vi "config_ini.vi"(11 "Path":path) -> ()   [LabVIEW 2013]
uses:
  <vilib>/Utility/config.llb/Read Key (Boolean).vi
  <vilib>/Utility/config.llb/Read Key (Double).vi
  FT_HMI.llb/GLOBAL_PUMPS_PARAMS.vi
  <vilib>/Utility/config.llb/NI_LVConfig.lvlib
panel:
  out "PUMPS_PARAMS":T1
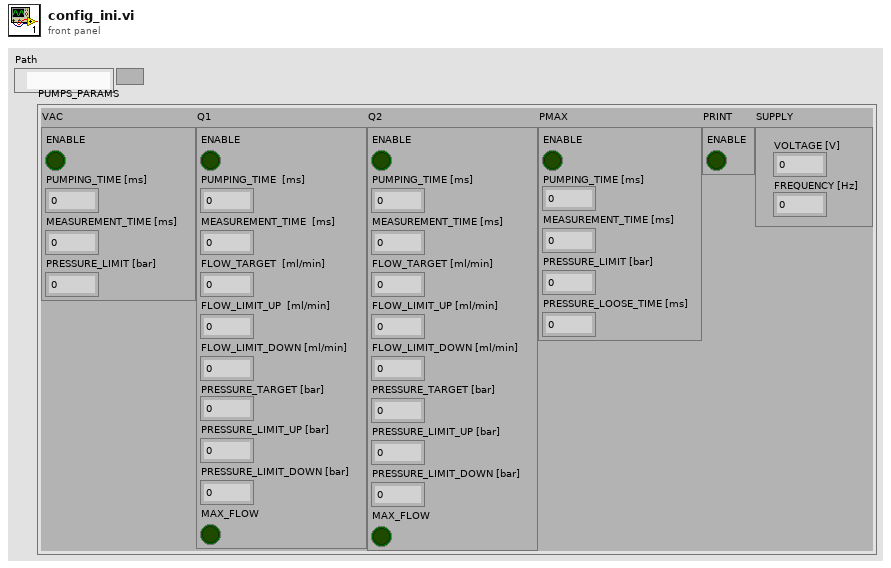
[diagram p1: front panel]
types:
  T1 = cluster{"VAC":cluster{"ENABLE":bool, "PUMPING_TIME [ms]":dbl, "MEASUREMENT_TIME [ms]":dbl, "PRESSURE_LIMIT [bar]":sgl}, "Q1":cluster{"ENABLE":bool, "PUMPING_TIME  [ms]":dbl, "MEASUREMENT_TIME  [ms]":sgl, "FLOW_TARGET  [ml/min]":sgl, "FLOW_LIMIT_UP  [ml/min]":sgl, "FLOW_LIMIT_DOWN [ml/min]":sgl, "PRESSURE_TARGET [bar]":sgl, "PRESSURE_LIMIT_UP [bar]":sgl, "PRESSURE_LIMIT_DOWN [bar]":sgl, "MAX_FLOW":bool}, "Q2":cluster{"ENABLE":bool, "PUMPING_TIME [ms]":dbl, "MEASUREMENT_TIME [ms]":dbl, "FLOW_TARGET [ml/min]":sgl, "FLOW_LIMIT_UP [ml/min]":sgl, "FLOW_LIMIT_DOWN [ml/min]":sgl, "PRESSURE_TARGET [bar]":sgl, "PRESSURE_LIMIT_UP [bar]":sgl, "PRESSURE_LIMIT_DOWN [bar]":sgl, "MAX_FLOW":bool}, "PMAX":cluster{"ENABLE":bool, "PUMPING_TIME [ms]":dbl, "MEASUREMENT_TIME [ms]":dbl, "PRESSURE_LIMIT [bar]":sgl, "PRESSURE_LOOSE_TIME [ms]":sgl}, "PRINT":cluster{"ENABLE":bool}, "SUPPLY":cluster{"VOLTAGE [V]":dbl, "FREQUENCY [Hz]":dbl}}
  T2 = typedef "NI_LVConfig.lvlib/Config Data RefNum.ctl" = refnum<k1>
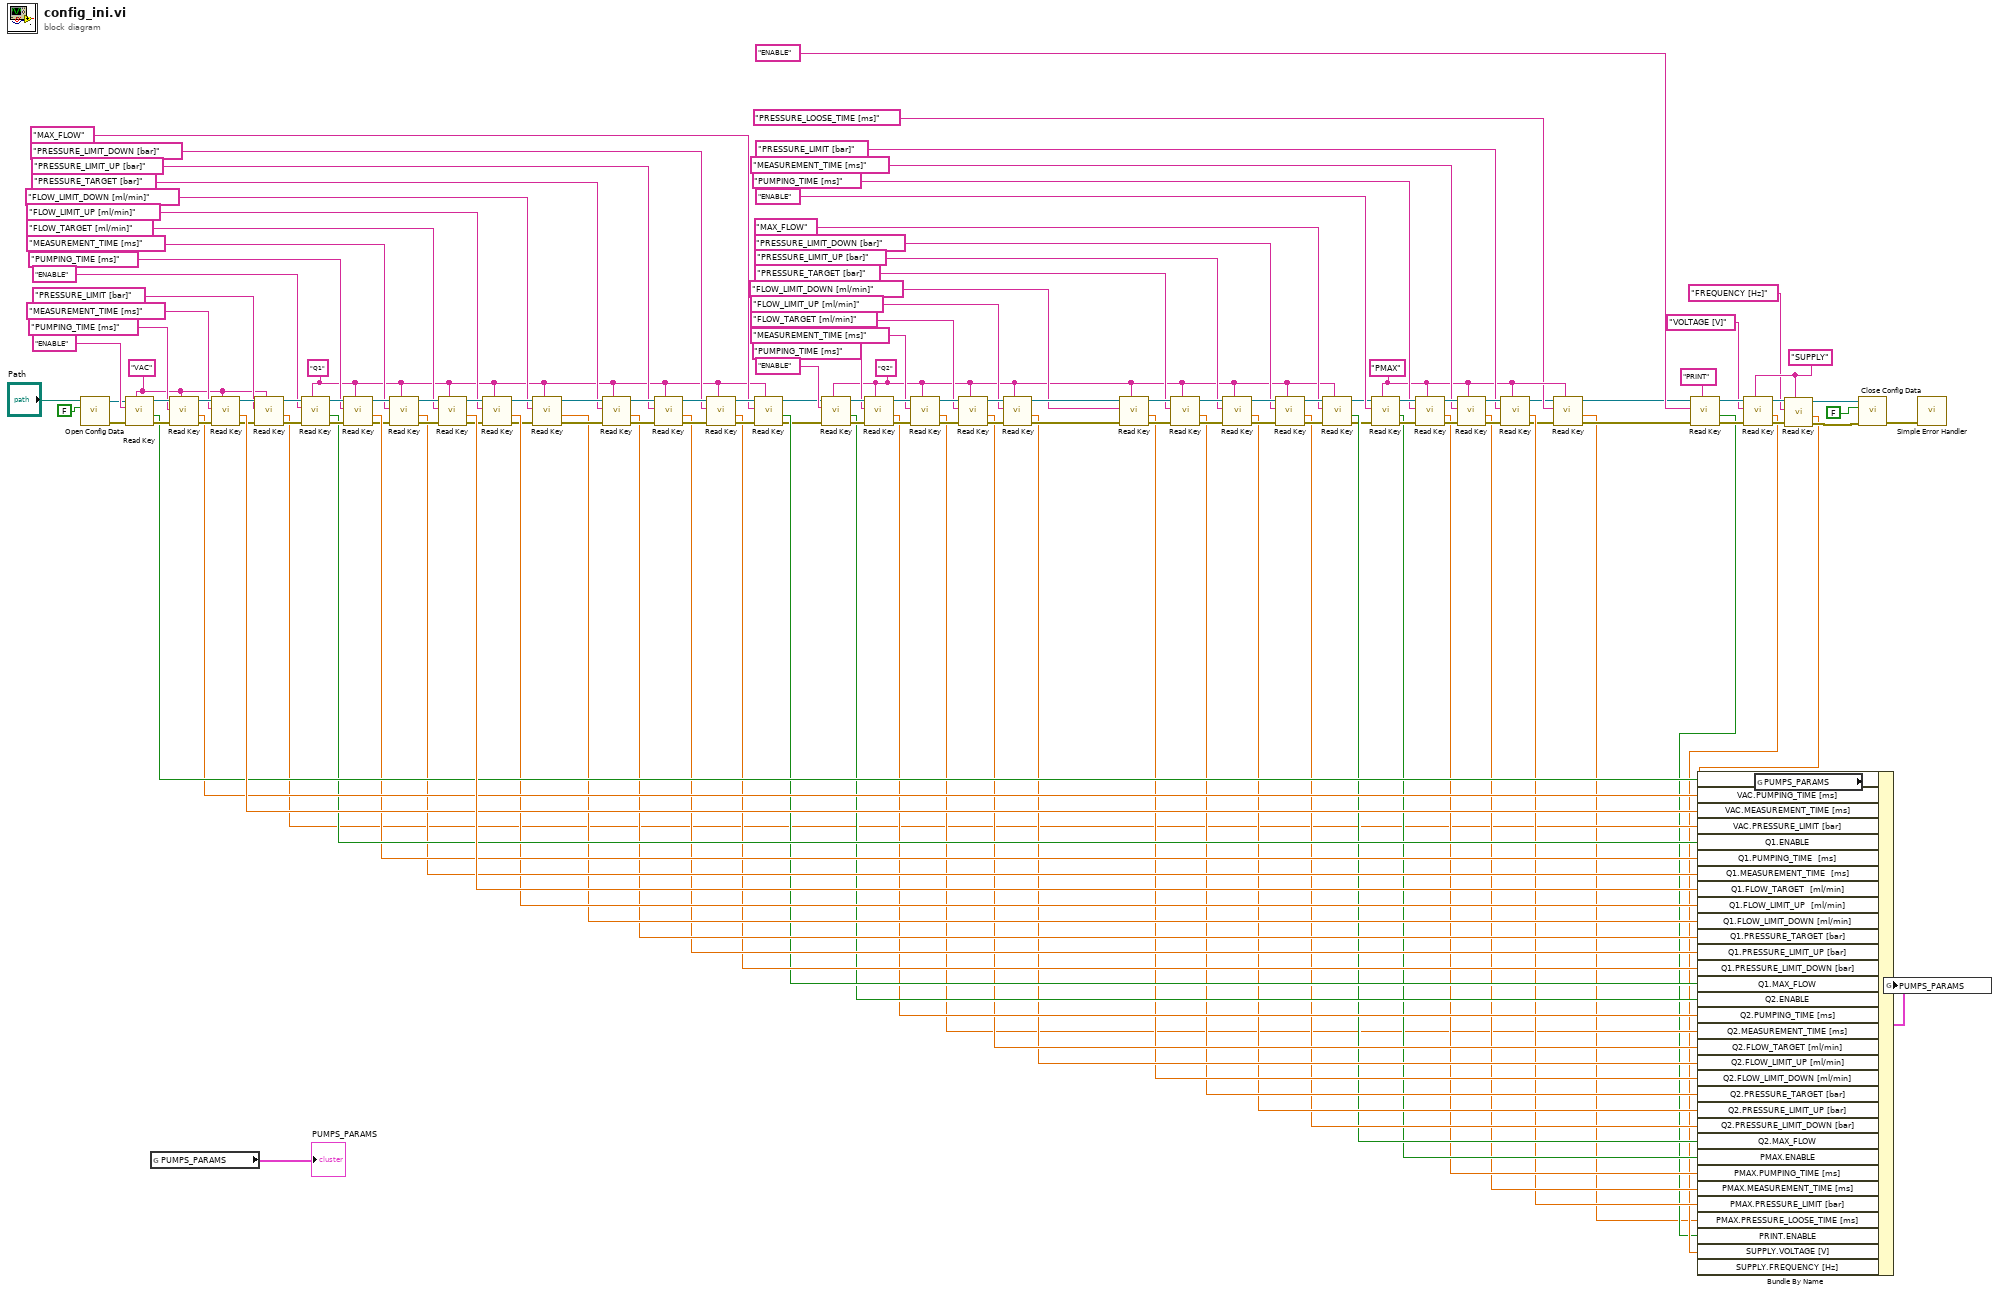
[diagram p0: block diagram]
diagram:
  w15 = "SUPPLY" ("section")
  w5 = "PMAX" ("section")
  w52 = "Q2" ("section")
  w81 = "Q1" ("section")
  w122 = "VAC" ("section")
  n1 = call <vilib>:"Open Config Data.vi"("create file if necessary (T)"=FALSE ("create file if necessary? (T)"), "configuration file path"="Path") -> ("error out"=w126:errorcluster, "refnum"=w125:T2)  [unwired: 7 in, 1 out]
  n2 = call-poly <vilib>:"Read Key.vi"("section"=w122, "error in (no error)"=w126, "key"="ENABLE" ("Key 1"), "refnum"=w125) -> ("error out"=w140:errorcluster, "value"=w116:bool, "refnum out"=w138:T2)  [unwired: 1 in, 4 out]
  n3 = global read "GLOBAL_PUMPS_PARAMS.vi" "PUMPS_PARAMS"() -> (→"PUMPS_PARAMS":T1)
  n4 = call-poly <vilib>:"Read Key.vi"("section"=w122, "error in (no error)"=w140, "key"="PUMPING_TIME [ms]" ("Key 2"), "refnum"=w138) -> ("error out"=w135:errorcluster, "value"=w115:dbl, "refnum out"=w136:T2)  [unwired: 1 in, 4 out]
  n5 = call-poly <vilib>:"Read Key.vi"("section"=w122, "error in (no error)"=w135, "key"="MEASUREMENT_TIME [ms]" ("Key 3"), "refnum"=w136) -> ("error out"=w139:errorcluster, "value"=w142:dbl, "refnum out"=w137:T2)  [unwired: 4 in, 1 out]
  n6 = call-poly <vilib>:"Read Key.vi"("section"=w122, "error in (no error)"=w139, "key"="PRESSURE_LIMIT [bar]" ("Key 4"), "refnum"=w137) -> ("error out"=w134:errorcluster, "value"=w11:dbl, "refnum out"=w133:T2)  [unwired: 2 in, 3 out]
  n7 = call-poly <vilib>:"Read Key.vi"("section"=w81, "error in (no error)"=w134, "key"="ENABLE" ("Key 5"), "refnum"=w133) -> ("error out"=w120:errorcluster, "value"=w114:bool, "refnum out"=w121:T2)  [unwired: 2 in, 3 out]
  n8 = call-poly <vilib>:"Read Key.vi"("section"=w81, "error in (no error)"=w120, "key"="PUMPING_TIME [ms]" ("Key 2"), "refnum"=w121) -> ("error out"=w107:errorcluster, "value"=w113:dbl, "refnum out"=w112:T2)  [unwired: 2 in, 3 out]
  n9 = call-poly <vilib>:"Read Key.vi"("section"=w81, "error in (no error)"=w107, "key"="MEASUREMENT_TIME [ms]" ("Key 3"), "refnum"=w112) -> ("error out"=w108:errorcluster, "value"=w103:dbl, "refnum out"=w111:T2)  [unwired: 2 in, 3 out]
  n10 = call-poly <vilib>:"Read Key.vi"("section"=w81, "error in (no error)"=w108, "key"="FLOW_TARGET [ml/min]" ("Key 3"), "refnum"=w111) -> ("error out"=w109:errorcluster, "value"=w143:dbl, "refnum out"=w110:T2)  [unwired: 2 in, 3 out]
  n11 = call-poly <vilib>:"Read Key.vi"("section"=w81, "error in (no error)"=w109, "key"="FLOW_LIMIT_UP [ml/min]" ("Key 3"), "refnum"=w110) -> ("error out"=w101:errorcluster, "value"=w102:dbl, "refnum out"=w96:T2)  [unwired: 2 in, 3 out]
  n12 = call-poly <vilib>:"Read Key.vi"("section"=w81, "error in (no error)"=w101, "key"="FLOW_LIMIT_DOWN [ml/min]" ("Key 3"), "refnum"=w96) -> ("error out"=w100:errorcluster, "value"=w86:dbl, "refnum out"=w95:T2)  [unwired: 2 in, 3 out]
  n13 = call-poly <vilib>:"Read Key.vi"("section"=w81, "error in (no error)"=w100, "key"="PRESSURE_TARGET [bar]" ("Key 3"), "refnum"=w95) -> ("error out"=w99:errorcluster, "value"=w85:dbl, "refnum out"=w94:T2)  [unwired: 2 in, 3 out]
  n14 = call-poly <vilib>:"Read Key.vi"("section"=w81, "error in (no error)"=w99, "key"="PRESSURE_LIMIT_UP [bar]" ("Key 3"), "refnum"=w94) -> ("error out"=w98:errorcluster, "value"=w84:dbl, "refnum out"=w93:T2)  [unwired: 2 in, 3 out]
  n15 = call-poly <vilib>:"Read Key.vi"("section"=w81, "error in (no error)"=w98, "key"="PRESSURE_LIMIT_DOWN [bar]" ("Key 3"), "refnum"=w93) -> ("error out"=w97:errorcluster, "value"=w83:dbl, "refnum out"=w92:T2)  [unwired: 2 in, 3 out]
  n16 = call-poly <vilib>:"Read Key.vi"("section"=w81, "error in (no error)"=w97, "key"="MAX_FLOW" ("Key 5"), "refnum"=w92) -> ("error out"=w51:errorcluster, "value"=w82:bool, "refnum out"=w50:T2)  [unwired: 2 in, 3 out]
  n17 = call-poly <vilib>:"Read Key.vi"("section"=w52, "error in (no error)"=w51, "key"="ENABLE" ("Key 5"), "refnum"=w50) -> ("error out"=w78:errorcluster, "value"=w49:bool, "refnum out"=w79:T2)  [unwired: 2 in, 3 out]
  n18 = call-poly <vilib>:"Read Key.vi"("section"=w52, "error in (no error)"=w78, "key"="PUMPING_TIME [ms]" ("Key 2"), "refnum"=w79) -> ("error out"=w71:errorcluster, "value"=w48:dbl, "refnum out"=w76:T2)  [unwired: 2 in, 3 out]
  n19 = call-poly <vilib>:"Read Key.vi"("section"=w52, "error in (no error)"=w71, "key"="MEASUREMENT_TIME [ms]" ("Key 3"), "refnum"=w76) -> ("error out"=w72:errorcluster, "value"=w13:dbl, "refnum out"=w75:T2)  [unwired: 2 in, 3 out]
  n20 = call-poly <vilib>:"Read Key.vi"("section"=w52, "error in (no error)"=w72, "key"="FLOW_TARGET [ml/min]" ("Key 3"), "refnum"=w75) -> ("error out"=w73:errorcluster, "value"=w47:dbl, "refnum out"=w74:T2)  [unwired: 2 in, 3 out]
  n21 = call-poly <vilib>:"Read Key.vi"("section"=w52, "error in (no error)"=w73, "key"="FLOW_LIMIT_UP [ml/min]" ("Key 3"), "refnum"=w74) -> ("error out"=w67:errorcluster, "value"=w46:dbl, "refnum out"=w62:T2)  [unwired: 2 in, 3 out]
  n22 = call-poly <vilib>:"Read Key.vi"("section"=w52, "error in (no error)"=w67, "key"="FLOW_LIMIT_DOWN [ml/min]" ("Key 3"), "refnum"=w62) -> ("error out"=w66:errorcluster, "value"=w45:dbl, "refnum out"=w61:T2)  [unwired: 2 in, 3 out]
  n23 = call-poly <vilib>:"Read Key.vi"("section"=w52, "error in (no error)"=w66, "key"="PRESSURE_TARGET [bar]" ("Key 3"), "refnum"=w61) -> ("error out"=w65:errorcluster, "value"=w44:dbl, "refnum out"=w60:T2)  [unwired: 2 in, 3 out]
  n24 = call-poly <vilib>:"Read Key.vi"("section"=w52, "error in (no error)"=w65, "key"="PRESSURE_LIMIT_UP [bar]" ("Key 3"), "refnum"=w60) -> ("error out"=w64:errorcluster, "value"=w43:dbl, "refnum out"=w59:T2)  [unwired: 2 in, 3 out]
  n25 = call-poly <vilib>:"Read Key.vi"("section"=w52, "error in (no error)"=w64, "key"="PRESSURE_LIMIT_DOWN [bar]" ("Key 3"), "refnum"=w59) -> ("error out"=w63:errorcluster, "value"=w42:dbl, "refnum out"=w58:T2)  [unwired: 2 in, 3 out]
  n26 = call-poly <vilib>:"Read Key.vi"("section"=w52, "error in (no error)"=w63, "key"="MAX_FLOW" ("Key 5"), "refnum"=w58) -> ("error out"=w24:errorcluster, "value"=w41:bool, "refnum out"=w23:T2)  [unwired: 2 in, 3 out]
  n27 = call-poly <vilib>:"Read Key.vi"("section"=w5, "error in (no error)"=w24, "key"="ENABLE" ("Key 1"), "refnum"=w23) -> ("error out"=w40:errorcluster, "value"=w30:bool, "refnum out"=w38:T2)  [unwired: 1 in, 4 out]
  n28 = call-poly <vilib>:"Read Key.vi"("section"=w5, "error in (no error)"=w40, "key"="PUMPING_TIME [ms]" ("Key 2"), "refnum"=w38) -> ("error out"=w35:errorcluster, "value"=w29:dbl, "refnum out"=w36:T2)  [unwired: 1 in, 4 out]
  n29 = call-poly <vilib>:"Read Key.vi"("section"=w5, "error in (no error)"=w35, "key"="MEASUREMENT_TIME [ms]" ("Key 3"), "refnum"=w36) -> ("error out"=w39:errorcluster, "value"=w28:dbl, "refnum out"=w37:T2)  [unwired: 4 in, 1 out]
  n30 = call-poly <vilib>:"Read Key.vi"("section"=w5, "error in (no error)"=w39, "key"="PRESSURE_LIMIT [bar]" ("Key 4"), "refnum"=w37) -> ("error out"=w1:errorcluster, "value"=w27:dbl, "refnum out"=w2:T2)  [unwired: 2 in, 3 out]
  n31 = call-poly <vilib>:"Read Key.vi"("section"=w5, "error in (no error)"=w1, "key"="PRESSURE_LOOSE_TIME [ms]" ("Key 4"), "refnum"=w2) -> ("error out"=w7:errorcluster, "value"=w3:dbl, "refnum out"=w6:T2)  [unwired: 2 in, 3 out]
  n32 = call-poly <vilib>:"Read Key.vi"("section"="PRINT", "error in (no error)"=w7, "key"="ENABLE" ("Key 5"), "refnum"=w6) -> ("error out"=w22:errorcluster, "value"=w8:bool, "refnum out"=w21:T2)  [unwired: 1 in, 4 out]
  n33 = call-poly <vilib>:"Read Key.vi"("section"=w15, "error in (no error)"=w22, "key"="VOLTAGE [V]" ("Key 4"), "refnum"=w21) -> ("error out"=w19:errorcluster, "value"=w9:dbl, "refnum out"=w17:T2)  [unwired: 4 in, 1 out]
  n34 = global read "GLOBAL_PUMPS_PARAMS.vi" "PUMPS_PARAMS"() -> (w118:T1)
  n35 = call-poly <vilib>:"Read Key.vi"("section"=w15, "error in (no error)"=w19, "key"="FREQUENCY [Hz]" ("Key 3"), "refnum"=w17) -> ("error out"=w18:errorcluster, "value"=w10:dbl, "refnum out"=w16:T2)  [unwired: 4 in, 1 out]
  n36 = Bundle By Name(cluster=w118, "VAC.ENABLE"=w116, "VAC.PUMPING_TIME [ms]"=w115, "VAC.MEASUREMENT_TIME [ms]"=w142, "VAC.PRESSURE_LIMIT [bar]"=w11, "Q1.ENABLE"=w114, "Q1.PUMPING_TIME  [ms]"=w113, "Q1.MEASUREMENT_TIME  [ms]"=w103, "Q1.FLOW_TARGET  [ml/min]"=w143, "Q1.FLOW_LIMIT_UP  [ml/min]"=w102, "Q1.FLOW_LIMIT_DOWN [ml/min]"=w86, "Q1.PRESSURE_TARGET [bar]"=w85, "Q1.PRESSURE_LIMIT_UP [bar]"=w84, "Q1.PRESSURE_LIMIT_DOWN [bar]"=w83, "Q1.MAX_FLOW"=w82, "Q2.ENABLE"=w49, "Q2.PUMPING_TIME [ms]"=w48, "Q2.MEASUREMENT_TIME [ms]"=w13, "Q2.FLOW_TARGET [ml/min]"=w47, "Q2.FLOW_LIMIT_UP [ml/min]"=w46, "Q2.FLOW_LIMIT_DOWN [ml/min]"=w45, "Q2.PRESSURE_TARGET [bar]"=w44, "Q2.PRESSURE_LIMIT_UP [bar]"=w43, "Q2.PRESSURE_LIMIT_DOWN [bar]"=w42, "Q2.MAX_FLOW"=w41, "PMAX.ENABLE"=w30, "PMAX.PUMPING_TIME [ms]"=w29, "PMAX.MEASUREMENT_TIME [ms]"=w28, "PMAX.PRESSURE_LIMIT [bar]"=w27, "PMAX.PRESSURE_LOOSE_TIME [ms]"=w3, "PRINT.ENABLE"=w8, "SUPPLY.VOLTAGE [V]"=w9, "SUPPLY.FREQUENCY [Hz]"=w10) -> (w117:T1)
  n37 = call <vilib>:"Close Config Data.vi"("error in (no error)"=w18, "write file if changed (T)"=FALSE ("write configuration file? (T)"), "refnum"=w16) -> ("error out"=w127:errorcluster)  [unwired: 8 out]
  n38 = global write "GLOBAL_PUMPS_PARAMS.vi" "PUMPS_PARAMS"(w117) -> ()
  n39 = call <vilib>:"Simple Error Handler.vi"("error in (no error)"=w127) -> ()  [unwired: 1 in, 8 out]
